vi "globalnyWspolrzedne.vi"() -> ()   [LabVIEW 2014]
uses:
  glownaMaszynaStanowVIs/wczytajListePunktowVIs/RodzajPomiarow.ctl
panel:
  out "Współrzędne w globalnym układzie":dbl[][][](array[numeric]) format="%#.2g"
  in  "r":dbl
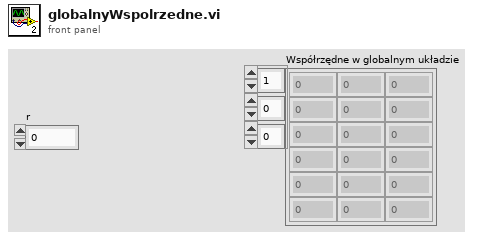
[diagram p1: front panel]
types:
  T1 = typedef "RodzajPomiarow.ctl" = enum16{"Izolacyjność Akustyczna ISO 10140", "Sekwencja testowa"}
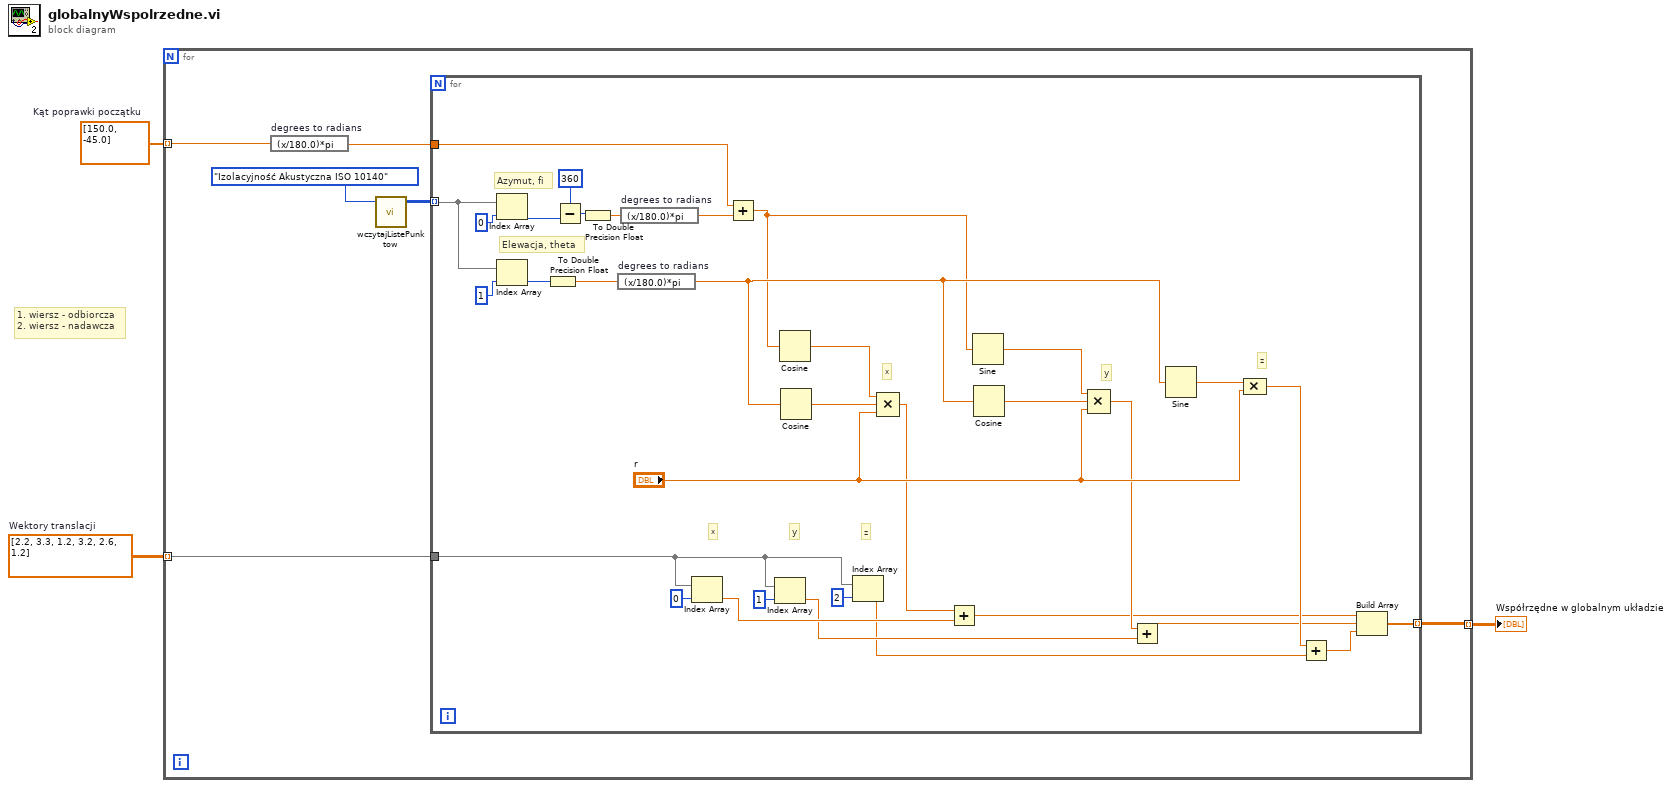
[diagram p0: block diagram]
diagram:
  w1 = dbl[] [150.0, -45.0]  # Kąt poprawki początku
  w3 = dbl[][] [[2.2, 3.3, 1.2], [3.2, 2.6, 1.2]]  # Wektory translacji
  # "1. wiersz - odbiorcza\n2. wiersz - nadawcza"
  n1 = for {
    tunnel: w3 -> [w7] mode=indexing
    tunnel: [w6] -> w2 mode=indexing
    tunnel: w1 -> [w5] mode=indexing
    n2 = expression code="(x/180.0)*pi" "degrees to radians"(w5) -> (w4:dbl)
    n3 = call "wczytajListePunktow.vi"("Rodzaj pomiarow"=RodzajPomiarow."Izolacyjność Akustyczna ISO 10140") -> ("Wspolrzedne katowe"=w8:i32[][])  [unwired: 4 in]
    n4 = for {
      tunnel: w8 -> [w40] mode=indexing
      tunnel: w7 -> [w32]
      tunnel: [w19] -> w6 mode=indexing
      tunnel: w4 -> [w13]
      # "z"
      # "y"
      # "x"
      # "z"
      # "y"
      # "x"
      # "Elewacja, theta"
      # "Azymut, fi"
      n5 = Index Array(array=w40, index=0) -> (element=w11:i32)
      n6 = Index Array(array=w40, index=1) -> (element=w39:i32)
      n7 = To Double Precision Float(number=w39) -> (double precision float=w17:dbl)
      n8 = Subtract(x=360, y=w11) -> (x-y=w12:i32)
      n9 = To Double Precision Float(number=w12) -> (double precision float=w18:dbl)
      n10 = expression code="(x/180.0)*pi" "degrees to radians"(w17) -> (w16:dbl)
      n11 = expression code="(x/180.0)*pi" "degrees to radians"(w18) -> (w15:dbl)
      n12 = Index Array(array=w32, index=0) -> (element=w27:dbl)
      n13 = Add(x=w13, y=w15) -> (x+y=w14:dbl)
      n14 = Index Array(array=w32, index=1) -> (element=w25:dbl)
      n15 = Cosine(x=w14) -> (cos(x)=w38:dbl)
      n16 = Cosine(x=w16) -> (cos(x)=w37:dbl)
      n17 = Index Array(array=w32, index=2) -> (element=w23:dbl)
      n18 = Compound Arithmetic op=MULTIPLY(w38, w37, "r") -> (w28:dbl)
      n19 = Add(x=w28, y=w27) -> (x+y=w22:dbl)
      n20 = Sine(x=w14) -> (sin(x)=w36:dbl)
      n21 = Cosine(x=w16) -> (cos(x)=w35:dbl)
      n22 = Compound Arithmetic op=MULTIPLY(w36, w35, "r") -> (w26:dbl)
      n23 = Add(x=w26, y=w25) -> (x+y=w21:dbl)
      n24 = Sine(x=w16) -> (sin(x)=w33:dbl)
      n25 = Compound Arithmetic op=MULTIPLY(w33, "r") -> (w24:dbl)
      n26 = Add(x=w24, y=w23) -> (x+y=w20:dbl)
      n27 = Build Array(w22, w21, w20) -> (w19:dbl[])
    }
  }
  "Współrzędne w globalnym układzie" <- w2
